vi "Annotations.vi"(11 "Input 1":dbl) -> (3 "Output 1":dbl)   [LabVIEW 2024]
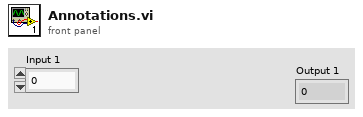
[diagram p1: front panel]
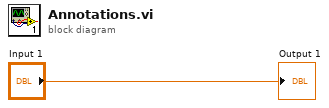
[diagram p0: block diagram]
diagram:
  "Output 1" <- "Input 1"
